vi "AI Callback 1 CPU.vi"(11 "IRQ Number":u8) -> ()   [LabVIEW 2021]
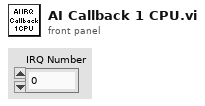
[diagram p1: front panel]
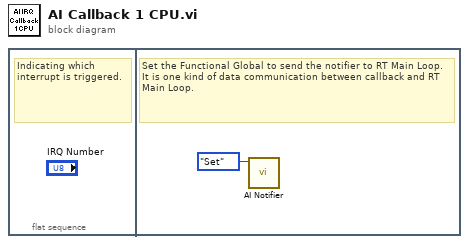
[diagram p0: block diagram]
diagram:
  n1 = flat-sequence {
    frame #0 {
      # "Indicating which interrupt is triggered."
    }
    frame #1 {
      # "Set the Functional Global to send the notifier to RT Main Loop. It is one kind of data communication between callback and RT Main Loop."
      n2 = call "AI Notifier.vi"("Action"=enum16{"Get", "Set"}."Set") -> ()  [unwired: 10 in, 1 out]
    }
  }
